vi "test matrix_int.vi"() -> ()   [LabVIEW 2012, in "LightPipes.lvlib"]
uses:
  Lightpipes.lvlib
panel:
  out "matrix out 2D":dbl[][](array[numeric])
  in  "n_grid":i32=128
  in  "Initial Beam":path=path "C:/Users/Tri Nguyen/Documents/lightpipes/LabView/beam images/final_beam.pgm"
  in  "c2":i16(ring) items=["subst", "mult"]
  in  "c1":i16(ring) items=["int", "pha"]
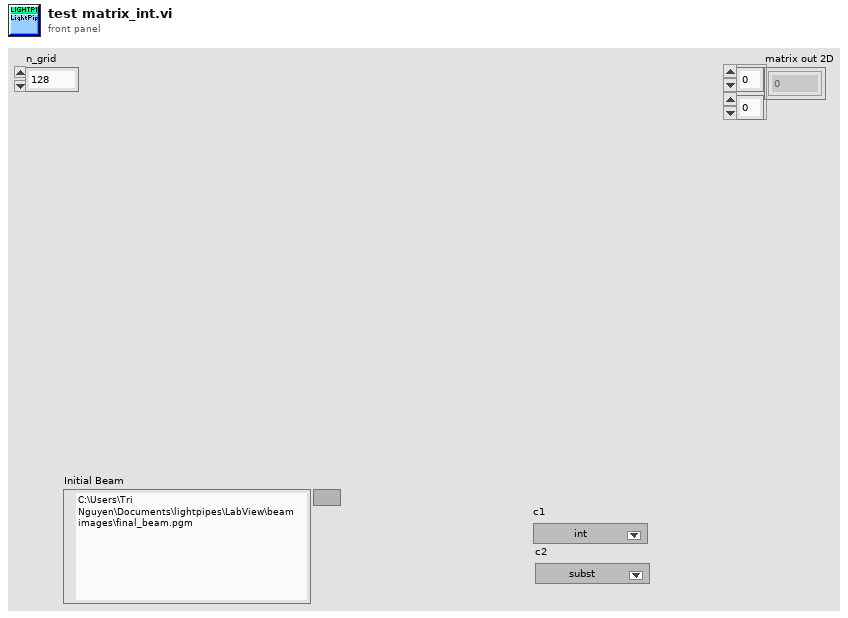
[diagram p1: front panel]
types:
  T1 = cluster{"n_grid":i32, "@dummy control@":i8, "@dummy control@":i8, "@dummy control@":i8, "@dummy control@":i8, "size":dbl, "lambda":dbl, "int1":i32, "int2":i32, "int3":i32, "@dummy control@":i8, "@dummy control@":i8, "@dummy control@":i8, "@dummy control@":i8, "double1":dbl, "double2":dbl, "double3":dbl, "real":u32, "imaginary":u32}
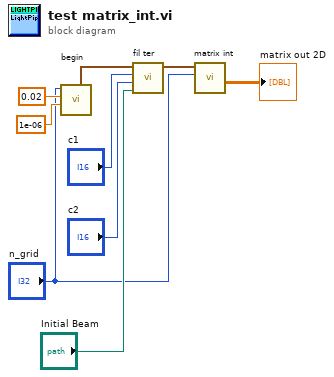
[diagram p0: block diagram]
diagram:
  n1 = call "begin.vi"("lambda"=1e-06, "size_grid"=0.02, "n_grid"="n_grid") -> ("field out"=w9:T1)  [unwired: 8 in]
  n2 = call "fil ter.vi"("Path"="Initial Beam", "multiplication/ substitution"="c2", "intensity / phase"="c1", "field"=w9) -> ("field out"=w5:T1)  [unwired: 6 in, 1 out]
  n3 = call "matrix int.vi"("n_grid"="n_grid", "field"=w5) -> ("matrix out 2D"=→"matrix out 2D":dbl[][])  [unwired: 8 in, 1 out]
